vi "PKG_IMC_GetPassword.vi"(9 "pwlen":string, 10 "password":string, 11 "handle":u32) -> (1 "pwlen out":string, 2 "password out":string, 3 "handle out":u32, 5 "function return":i32)   [LabVIEW 2011, in "IMC_Pkg4xxx.lvlib"]
doc: "PKG_IMC_GetPassword(IMC_HANDLE handle, char password[128], char *pwlen);"
uses:
  IMC_Pkg4xxx.lvlib
  IMC_Pkg4xxx.dll
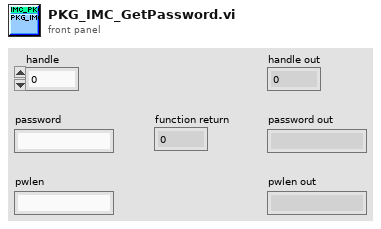
[diagram p1: front panel]
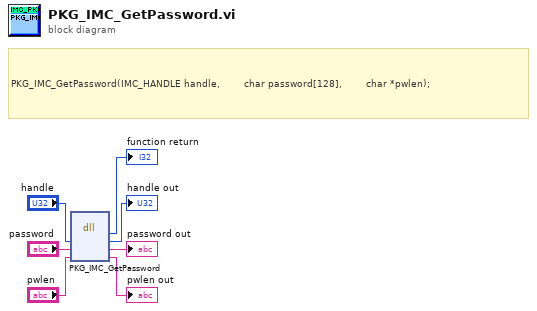
[diagram p0: block diagram]
diagram:
  # "PKG_IMC_GetPassword(IMC_HANDLE handle,  \t\t\t\t\t\tchar password[128],\t\t\t\t\t\t\t\tchar *pwlen);"
  n1 = dll-call lib="PTH1mabs F光盘刻录\niMC MotionIMCNet_V4.0IMCAppincLabviewIMC_PKG4xxxIMC_PKG4xxx\nIMC_Pkg4xxx.*" fn="PKG_IMC_GetPassword"("handle"="handle", "password"="password", "pwlen"="pwlen") -> (→"function return":i32, "handle"=→"handle out":u32, "password"=→"password out":string, "pwlen"=→"pwlen out":string)  [unwired: 3 in, 2 out]
